vi "Create promotion move.vi"(9 "Promotion type":T1, 10 "Destination":T2={"File"=enum."d", "Rank"=enum."4"}, 11 "Source":T2={"File"=enum."d", "Rank"=enum."4"}) -> (3 "Promotion out":refnum<class "Promotion.lvclass">)   [LabVIEW 2015, in "Chesslib.lvlib" / "Promotion.lvclass"]
uses:
  Promotion.lvclass
  typedef/Square.ctl
  typedef/File.ctl
  typedef/Rank.ctl
  typedef/Piece type.ctl
  Promotion.lvclass/Promotion.ctl
  Move/Move.lvclass
  Chesslib.lvlib
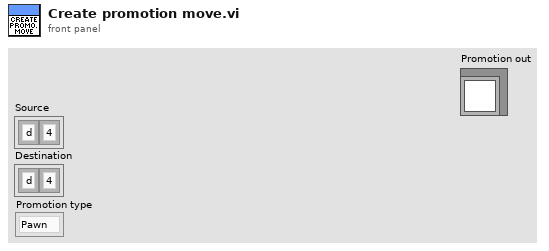
[diagram p1: front panel]
types:
  T1 = typedef "Chesslib.lvlib/Piece type.ctl" = enum16{"Pawn", "Bishop", "Knight", "Rook", "Queen", "King"}
  T2 = typedef "Chesslib.lvlib/Square.ctl" = cluster{"File":T3, "Rank":T4}
  T3 = typedef "Chesslib.lvlib/File.ctl" = enum8{"a", "b", "c", "d", "e", "f", "g", "h"}
  T4 = typedef "Chesslib.lvlib/Rank.ctl" = enum8{"1", "2", "3", "4", "5", "6", "7", "8"}
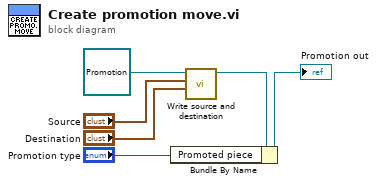
[diagram p0: block diagram]
diagram:
  n1 = call "Write source and destination.vi"("Destination"="Destination", "Source"="Source", "Move in"=refnum<class "Promotion.lvclass"> refnum ("Promotion in")) -> ("Move out"=w5:refnum<class "Promotion.lvclass">)  [unwired: 8 in]
  n2 = Bundle By Name(cluster=w5, "Promoted piece"="Promotion type") -> (→"Promotion out":refnum<class "Promotion.lvclass">)
